vi "Create Camera Map Queue.vi"(7 "Action":enum16{"Read", "Write"}(ring), 10 "Image in":T1, 11 "Camera":string) -> (1 "key not found?":bool, 2 "Image out":T1)   [LabVIEW 2025]
uses:
  <vilib>/vision/Image Controls.llb/IMAQ Image.ctl
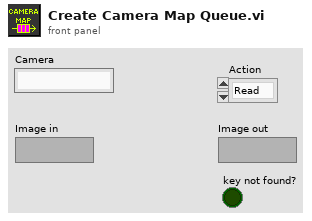
[diagram p1: front panel]
types:
  T1 = typedef "IMAQ Image.ctl" = refnum<image>
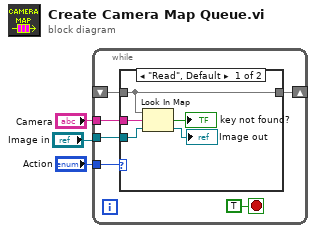
[diagram p0: block diagram]
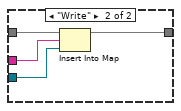
[diagram p2: hidden frame]
diagram:
  n1 = while {
    shift-right: [w7] -> _
    shift-left: _ -> [w8]
    tunnel: "Camera" -> [w6]
    tunnel: "Image in" -> [w5]
    tunnel: "Action" -> [w4]
    stop <- TRUE stop-if-true
    n2 = case shown="\"Read\", Default" w4 {
      tunnel: w8 -> [w13 w18]
      tunnel: w6 -> [w11 w16]
      tunnel: w5 -> [w14 w15]
      tunnel: [w13 w17] -> w7
      frame "Read", Default {
        n3 = Look In Map(map=w13, key=w11, default value=w14) -> (key not found?=→"key not found?":bool, value=→"Image out":T1)
      }
      frame "Write" {
        n4 = Insert Into Map(map in=w18, key=w16, value=w15) -> (map out=w17:map{string, T1})  [unwired: 2 out]
      }
    }
  }
